vi "Translation2d_Create_DistAng.vi"(10 "Angle":T1={"VALUE"=0.0, "COS"=1.0, "SIN"=0.0} {"SIN" format="%13.4f"; "COS" format="%13.4f"; "VALUE" format="%13.4f"}, 11 "Dist":dbl) -> (3 "TRANSLATION":T2 {"Y" format="%14.3f"; "X" format="%14.3f"})   [LabVIEW 2019, in "Trajectory_Library.lvlib"]
doc: "Constructs a Translation2d with the provided distance and angle. This is essentially converting from polar coordinates to Cartesian coordinates.\n\nRepresents a translation in 2d space. This object can be used to represent a point or a vector.\n\nThis assumes that you are using conventional mathematical axes. When the robot is placed on the origin, facing toward the X direction, moving forward increases the X, whereas moving to the left increases the Y.\n\nParameters:\n - Dist - Distance.\n - Ang - Rotation representing the angle.\n\nReturns\n - TRANSLATION - The TRANSLATION data structure"
uses:
  Trajectory_Library.lvlib
  TRANSLATION2D.ctl
  ROTATION2D.ctl
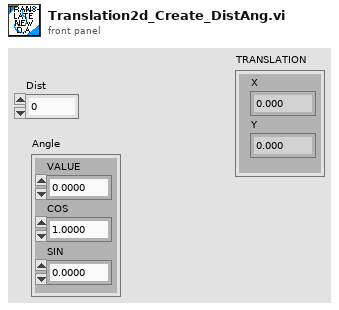
[diagram p1: front panel]
types:
  T1 = typedef "Trajectory_Library.lvlib/ROTATION2D.ctl" = cluster{"VALUE":dbl, "COS":dbl, "SIN":dbl}
  T2 = typedef "Trajectory_Library.lvlib/TRANSLATION2D.ctl" = cluster{"X":dbl, "Y":dbl}
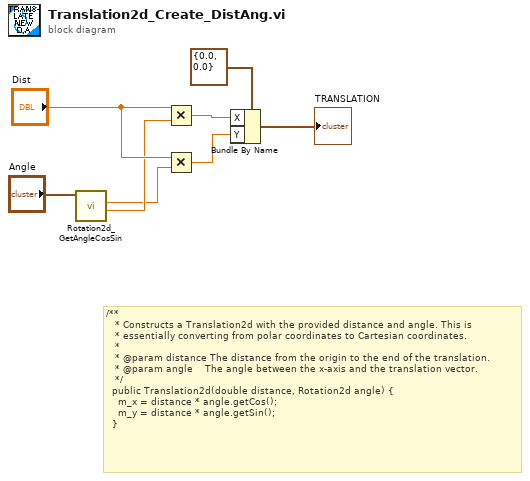
[diagram p0: block diagram]
diagram:
  # "/**\n   * Constructs a Translation2d with the provided distance and angle. This is\n   * essentially converting from polar coordinates to Cartesian coordinates.\n   *\n   * @param distance The distance from the origin to the end of the translation.\n   * @param angle    The angle between the x-axis and the translation vector.\n   */\n  public Translation2d(double distance, Rotation2d angle) {\n    m_x = distance * angle.getCos();\n    m_y = distance * angle.getSin();\n  }"
  n1 = call "Rotation2d_GetAngleCosSin.vi"("in ROTATION"="Angle") -> ("Cosine"=w2:dbl, "Sine"=w1:dbl)  [unwired: 8 in, 1 out]
  n2 = Multiply(x="Dist", y=w2) -> (x*y=w4:dbl)
  n3 = Multiply(x="Dist", y=w1) -> (x*y=w3:dbl)
  n4 = Bundle By Name(cluster=T2 {"X"=0.0, "Y"=0.0} ("TRANSLATION"), "X"=w4, "Y"=w3) -> (→"TRANSLATION":T2)
